vi "bang_bang_controller_ElevatorSim_example.vi"() -> ()   [LabVIEW 2019]
uses:
  <vilib>/Rock Robotics/WPI/ThirdParty/JAS_Junk/TrajLib/BangBang_AtSetpoint.vi
  <vilib>/Rock Robotics/WPI/ThirdParty/JAS_Junk/TrajLib/BangBang_New.vi
  <vilib>/Rock Robotics/WPI/ThirdParty/JAS_Junk/TrajLib/BangBang_Calculate_SP_PV.vi
  <vilib>/Rock Robotics/WPI/ThirdParty/JAS_Junk/TrajLib/Trajectory_Library.lvlib
panel:
  out "AtSetpoint":bool
  in  "At Setpoint\nTolerance":dbl=0.1 min=0.0 max=4.0 step=0.025 format="%#_13g"
  in  "GO DOWN":bool
  out "Battery Voltage":dbl format="%20.3f"
  out "CO, Voltage, Current Chart":T1(graph)
  in  "GO UP":bool
  out "Elevator\nHeight \nSetpoint(SP)":dbl(slide) scale=-1.0..6.0
  out "Elevator\nHeight (PV)":dbl(slide) scale=-1.0..6.0
  out "SP, PV Chart":T2(graph)
  out "Motor Dmd (CO)":dbl format="%20.3f"
  out "Top\nReached":bool
  out "Bottom\nReached":bool
  out "Motor Amps":dbl format="%20.3f"
  # "Bang Bang Control of a simulated elevator"
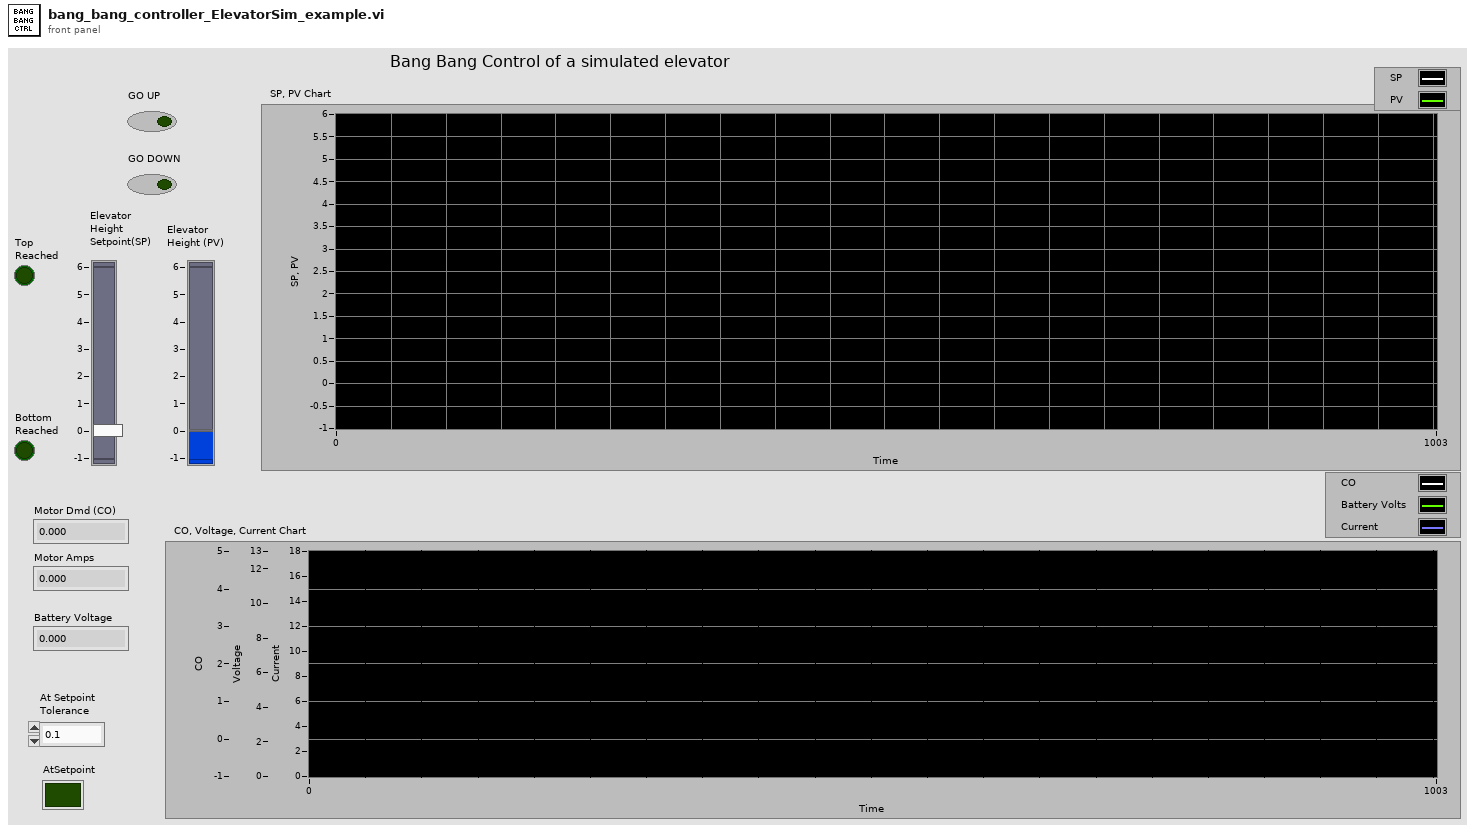
[diagram p1: front panel]
types:
  T1 = cluster{"ControlOutput":dbl, "Loaded Voltage":dbl, "Current":dbl}
  T2 = cluster{"Position_Meters":dbl, "Real Matrix Element":dbl}
  T3 = typedef "Trajectory_Library.lvlib/ELEVATOR_SIM.ctl" = cluster{"LinearSystemSim":T4, "GearBox":T7, "Gearing":dbl, "DrumRadius_M":dbl, "MinHeight_M":dbl, "MaxHeight_M":dbl, "CarriageMass_Kg":dbl, "SimulateGravity":bool}
  T4 = typedef "Trajectory_Library.lvlib/LINEAR_SYSTEM_SIM.ctl" = cluster{"m_Plant":T5, "m_X":T6, "m_Y":T6, "m_U":T6, "MeasureStdDev":T6}
  T5 = typedef "Trajectory_Library.lvlib/LINEAR_SYSTEM.ctl" = cluster{"m_A":T6, "m_B":T6, "m_C":T6, "m_D":T6, "States":i32, "Inputs":i32, "Outputs":i32}
  T6 = typedef "NI_Matrix.lvlib/RealMatrix.ctl" = dbl[][]
  T7 = typedef "Trajectory_Library.lvlib/DCMOTOR.CTL" = cluster{"nominalVoltage_Volts":dbl, "StallTorque_NM":dbl, "StallCurrent_Amps":dbl, "FreeCurrent_Amps":dbl, "FreeSpeed_RadPerSec":dbl, "R_Ohms":dbl, "KvINV_RadPerSecPerVolt":dbl, "Kt_NMPerAmp":dbl, "L_H":dbl, "Jr_KgM2":dbl}
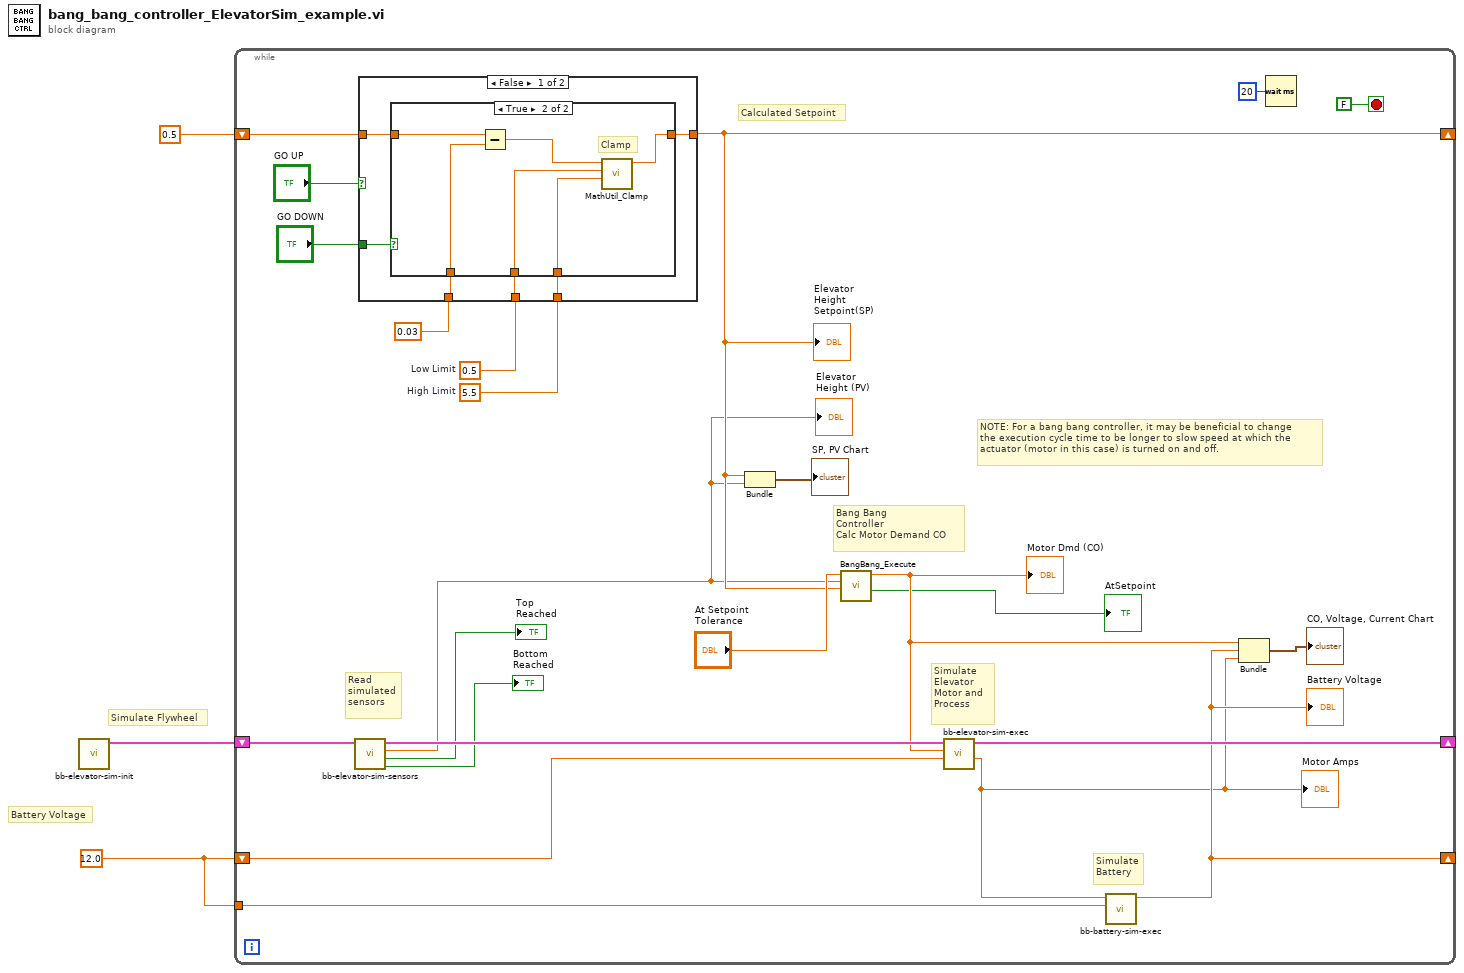
[diagram p0: block diagram]
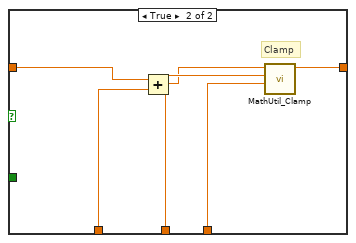
[diagram p3: hidden frame]
diagram:
  w3 = 12.0
  # "Simulate Flywheel"
  # "Battery Voltage"
  n1 = call "bb-elevator-sim-init.vi"() -> ("ElevatorSim"=w2:T3)  [unwired: 11 in]
  n2 = while {
    shift-right: [w23] -> _
    shift-left: w2 -> [w15]
    shift-right: [w11] -> _
    shift-left: w3 -> [w10]
    tunnel: w3 -> [w9]
    shift-right: [w7] -> _
    shift-left: 0.5 -> [w18]
    stop <- FALSE stop-if-true
    w20 = 5.5  # High Limit
    w19 = 0.5  # Low Limit
    # "NOTE: For a bang bang controller, it may be beneficial to change\nthe execution cycle time to be longer to slow speed at which the\nactuator (motor in this case) is turned on and off."
    # "Calculated Setpoint"
    # "Simulate\nBattery"
    # "Simulate \nElevator\nMotor and \nProcess"
    # "Bang Bang\nController\nCalc Motor Demand CO"
    # "Read\nsimulated\nsensors"
    n3 = call "bb-elevator-sim-sensors.vi"("inElevatorSim"=w15) -> ("AtLowLimit"=→"Bottom\nReached":bool, "At HIgh LImit"=→"Top\nReached":bool, "Height"=w6:dbl, "outElevatorSim"=w14:T3)  [unwired: 7 in]
    "Elevator\nHeight (PV)" <- w6
    n4 = case shown="False" "GO UP" {
      tunnel: w20 -> [w33 w46]
      tunnel: w19 -> [w32 w45]
      tunnel: w18 -> [w31 w42]
      tunnel: [w30 w44] -> w7
      tunnel: 0.03 ("y") -> [w29 w41]
      tunnel: "GO DOWN" -> [w28 _]
      frame False {
        n5 = case shown="True" w28 {
          tunnel: w33 -> [_ w39]
          tunnel: w32 -> [_ w38]
          tunnel: w31 -> [w34 w37]
          tunnel: [w34 w36] -> w30
          tunnel: w29 -> [_ w35]
          frame False {
          }
          frame True {
            # "Clamp"
            n6 = Subtract(x=w37, y=w35) -> (x-y=w40:dbl)
            n7 = call <vilib>:"MathUtil_Clamp.vi"("High Limit"=w39, "Low Limit"=w38, "Value"=w40) -> ("Result"=w36:dbl)  [unwired: 8 in]
          }
        }
      }
      frame True {
        # "Clamp"
        n8 = Add(x=w42, y=w41) -> (x+y=w43:dbl)
        n9 = call <vilib>:"MathUtil_Clamp.vi"("High Limit"=w46, "Low Limit"=w45, "Value"=w43) -> ("Result"=w44:dbl)  [unwired: 8 in]
      }
    }
    "Elevator\nHeight \nSetpoint(SP)" <- w7
    n10 = Bundle("Result"=w7, "Height"=w6) -> (→"SP, PV Chart":cluster{"Result":dbl, "Height":dbl})  [unwired: 1 in]
    n11 = call <vilib>:"BangBang_Execute.vi"("Setpoint"=w7, "Measurment"=w6, "Tolerance"="At Setpoint\nTolerance") -> ("AtSetpoint"=→"AtSetpoint":bool, "ControlOutput"=w8:dbl)  [unwired: 6 in, 1 out]
    "Motor Dmd (CO)" <- w8
    n12 = call "bb-elevator-sim-exec.vi"("Battery Voltage"=w10, "Motor Dmd CO"=w8, "inElevatorSim"=w14) -> ("Current"=w5:dbl, "out ElevatorSim"=w23:T3)  [unwired: 7 in]
    "Motor Amps" <- w5
    n13 = call "bb-battery-sim-exec.vi"("Nominal Battery\nVoltage"=w9, "Current Amps"=w5) -> ("Loaded Voltage"=w11:dbl)  [unwired: 9 in]
    "Battery Voltage" <- w11
    n14 = Bundle("ControlOutput"=w8, "Loaded Voltage"=w11, "Current"=w5) -> (→"CO, Voltage, Current Chart":T1)  [unwired: 1 in]
    n15 = Wait (ms)(milliseconds to wait=u32 20) -> ()  [unwired: 1 out]
  }
